vi "Sr830 VisaRW.vi"(0 "VISA Rsrc":refnum<visa-resource-name>="SR530", 2 "EOS (Aucun)":string, 3 "Délais (0 ms)":u32, 5 "ChaineCom":string caption="Chaîne de commande", 7 "Nbcomm":i32=1 caption="Nombre de \nCommandes", 9 "Nbcaract":u32=100 caption="Nombre de \ncaractères à lire", 11 "error in (no error)":errorcluster, 12 "Lecture?(T)":bool=TRUE) -> (4 "VISA Rsrc Out":refnum<visa-resource-name>="GPIB0::12::INSTR", 6 "ChaineRep":string caption="Chaîne de réponse", 14 "Count out":u32=44 caption="Nombre de caractères lus", 15 "error out":errorcluster)   [LabVIEW 2019]
doc: "Ce VI envoie des commande d'écriture et de lecture VISA à l'appareil GPIB. Il permet de ne pas séparer un question de sa réponse. Pour que cela fonctionne toute lecture d'un instrument doit se faire par ce VI."
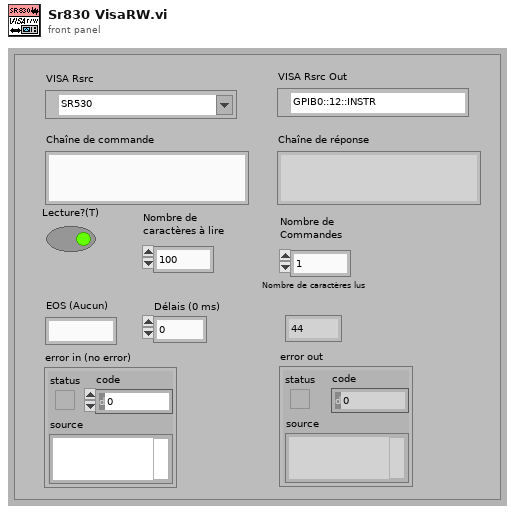
[diagram p1: front panel]
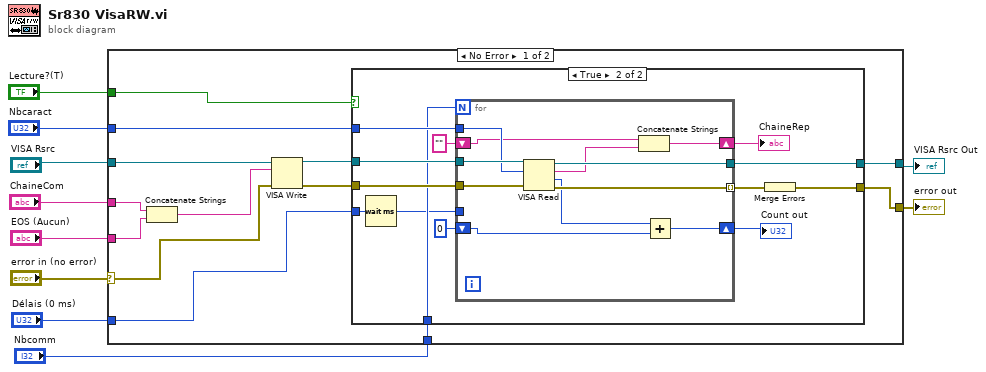
[diagram p0: block diagram]
diagram:
  n1 = case shown="No Error" "error in (no error)" {
    selector: "error in (no error)" -> [w17 w51]
    tunnel: "VISA Rsrc" -> [w18 w50]
    tunnel: [w23 w50] -> w2
    tunnel: "ChaineCom" -> [w22 _]
    tunnel: "EOS (Aucun)" -> [w21 _]
    tunnel: "Délais (0 ms)" -> [w14 _]
    tunnel: "Nbcaract" -> [w13 _]
    tunnel: "Lecture?(T)" -> [w12 _]
    tunnel: [w19 w51] -> w4
    tunnel: "Nbcomm" -> [w11 _]
    frame No Error {
      n2 = Concatenate Strings(w22, w21) -> (w20:string)
      n3 = VISA Write(VISA resource name=w18, write buffer=w20, error in (no error)=w17) -> (VISA resource name out=w16:refnum<visa-resource-name>, error out=w15:errorcluster)  [unwired: 1 out]
      n4 = case shown="True" w12 {
        tunnel: w16 -> [w25 w38]
        tunnel: [w25 w37] -> w23
        tunnel: w15 -> [w24 w36]
        tunnel: [w24 w26] -> w19
        tunnel: w13 -> [_ w34]
        tunnel: w14 -> [_ w33]
        tunnel: w11 -> [_ w32]
        frame False {
        }
        frame True {
          n5 = Wait (ms)(milliseconds to wait=w33) -> (millisecond timer value=w31:u32)
          n6 = for {
            N: w32 -> [_]
            tunnel: w38 -> [w49]
            tunnel: [w48] -> w37
            tunnel: w36 -> [w47]
            tunnel: [w46] -> w35 mode=indexing
            tunnel: w34 -> [w45]
            tunnel: w31 -> [_]
            shift-right: [w43] -> w29
            shift-left: "" -> [w42]
            shift-right: [w40] -> w27
            shift-left: u32 0 -> [w39]
            n7 = VISA Read(VISA resource name=w49, byte count=w45, error in (no error)=w47) -> (VISA resource name out=w48:refnum<visa-resource-name>, read buffer=w44:string, return count=w41:u32, error out=w46:errorcluster)
            n8 = Concatenate Strings(w42, w44) -> (w43:string)
            n9 = Add(x=w41, y=w39) -> (x+y=w40:u32)
          }
          "ChaineRep" <- w29
          "Count out" <- w27
          n10 = Merge Errors(w35) -> (w26:errorcluster)
        }
      }
    }
    frame Error {
    }
  }
  "error out" <- w4
  "VISA Rsrc Out" <- w2
